vi "States 2 Leds.vi"(10 "MixedModeStates":T1) -> (2 "Mixed Mode State Display":T2)   [LabVIEW 2013]
uses:
  Mixed Mode State Display.ctl
  MixedMode/Mixed Mode States.ctl
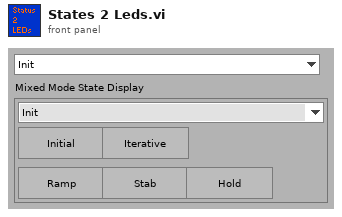
[diagram p1: front panel]
types:
  T1 = typedef "Mixed Mode States.ctl" = enum16{"Init", "Wait For DAQ", "Idle", "Start Initial Position", "Initial Position", "Start Initial Ramp", "Run Initial Ramp", "Start Iterative Stage", "Convergence Check", "Update Stiffness Jacobian", "Update Command", "Start Iterative Ramp", "Run Iterative Ramp", "Start Iterative Stabilize", "Iterative Stabilize", "Start Iterative Holding", "Iterative Holding", "Start Stabilize", "Stabilize", "Start Hold", "Holding", "Done", "Aborting", "Exit", "Nop"}
  T2 = typedef "Mixed Mode State Display.ctl" = cluster{"MixedModeStates":T1, "Initial":bool, "Iterative":bool, "Ramp":bool, "Stab":bool, "Hold":bool}
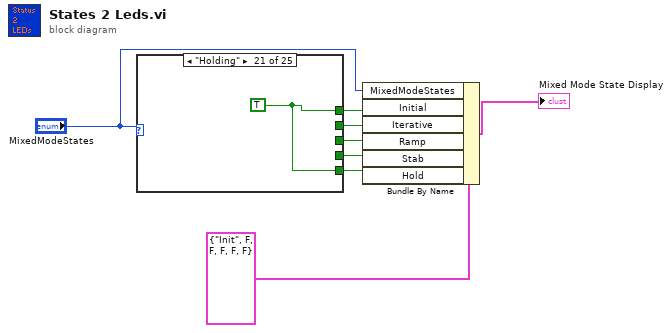
[diagram p0: block diagram]
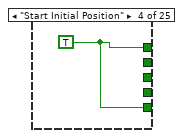
[diagram p5: hidden frame]
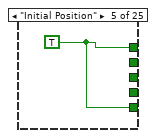
[diagram p6: hidden frame]
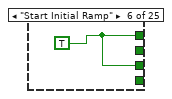
[diagram p7: hidden frame]
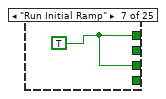
[diagram p8: hidden frame]
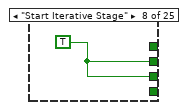
[diagram p9: hidden frame]
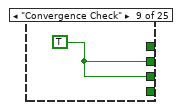
[diagram p10: hidden frame]
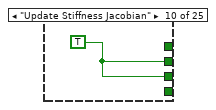
[diagram p11: hidden frame]
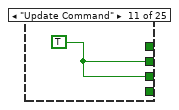
[diagram p12: hidden frame]
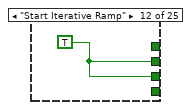
[diagram p13: hidden frame]
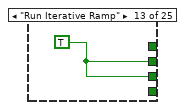
[diagram p14: hidden frame]
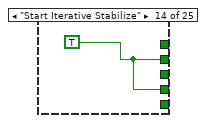
[diagram p15: hidden frame]
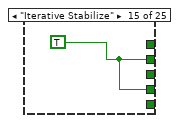
[diagram p16: hidden frame]
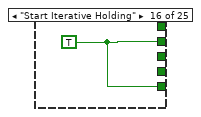
[diagram p17: hidden frame]
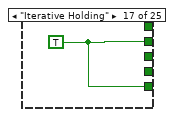
[diagram p18: hidden frame]
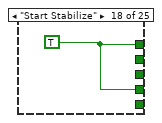
[diagram p19: hidden frame]
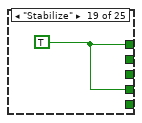
[diagram p20: hidden frame]
diagram:
  n1 = case shown="\"Holding\"" "MixedModeStates" {
    tunnel: [_ _ _ w9 w10 w11 w12 _ _ _ _ _ _ _ _ _ _ w23 w24 w25 w26 _ _ _ _] -> w5
    tunnel: [_ _ _ _ _ w11 w12 w13 w14 w15 w16 w17 w18 _ _ _ _ _ _ _ _ _ _ _ _] -> w4
    tunnel: [_ _ _ _ _ _ _ w13 w14 w15 w16 w17 w18 w19 w20 w21 w22 _ _ _ _ _ _ _ _] -> w3
    tunnel: [_ _ _ _ _ _ _ _ _ _ _ _ _ w19 w20 _ _ w23 w24 _ _ _ _ _ _] -> w2
    tunnel: [_ _ _ w9 w10 _ _ _ _ _ _ _ _ _ _ w21 w22 _ _ w25 w26 _ _ _ _] -> w1
    frame "Init" {
    }
    frame "Wait For DAQ" {
    }
    frame "Idle" {
    }
    frame "Start Initial Position" {
      w9 = TRUE
    }
    frame "Initial Position" {
      w10 = TRUE
    }
    frame "Start Initial Ramp" {
      w11 = TRUE
    }
    frame "Run Initial Ramp" {
      w12 = TRUE
    }
    frame "Start Iterative Stage" {
      w13 = TRUE
    }
    frame "Convergence Check" {
      w14 = TRUE
    }
    frame "Update Stiffness Jacobian" {
      w15 = TRUE
    }
    frame "Update Command" {
      w16 = TRUE
    }
    frame "Start Iterative Ramp" {
      w17 = TRUE
    }
    frame "Run Iterative Ramp" {
      w18 = TRUE
    }
    frame "Start Iterative Stabilize" {
      w19 = TRUE
    }
    frame "Iterative Stabilize" {
      w20 = TRUE
    }
    frame "Start Iterative Holding" {
      w21 = TRUE
    }
    frame "Iterative Holding" {
      w22 = TRUE
    }
    frame "Start Stabilize" {
      w23 = TRUE
    }
    frame "Stabilize" {
      w24 = TRUE
    }
    frame "Start Hold" {
      w25 = TRUE
    }
    frame "Holding" {
      w26 = TRUE
    }
    frame "Done" {
    }
    frame "Aborting" {
    }
    frame "Exit" {
    }
    frame "Nop" {
    }
  }
  n2 = Bundle By Name(cluster=T2 {"MixedModeStates"=enum."Init", "Initial"=FALSE, "Iterative"=FALSE, "Ramp"=FALSE, "Stab"=FALSE, "Hold"=FALSE} ("Mixed Mode State Display"), "MixedModeStates"="MixedModeStates", "Initial"=w5, "Iterative"=w3, "Ramp"=w4, "Stab"=w2, "Hold"=w1) -> (→"Mixed Mode State Display":T2)
